vi "shiftregister&graphs.vi"() -> ()   [LabVIEW 2020]
panel:
  out "Waveform Graph":dbl[](graph)
  out "Waveform Chart":dbl(graph)
  in  "stop":bool
  out "Numeric 2":i64
  out "Numeric":i64
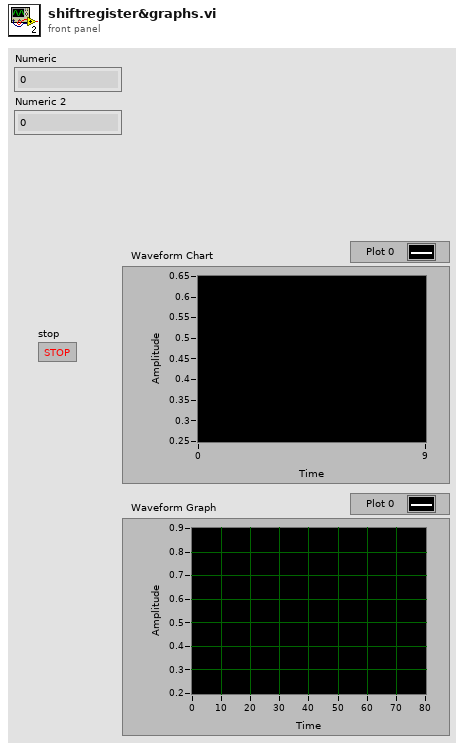
[diagram p1: front panel]
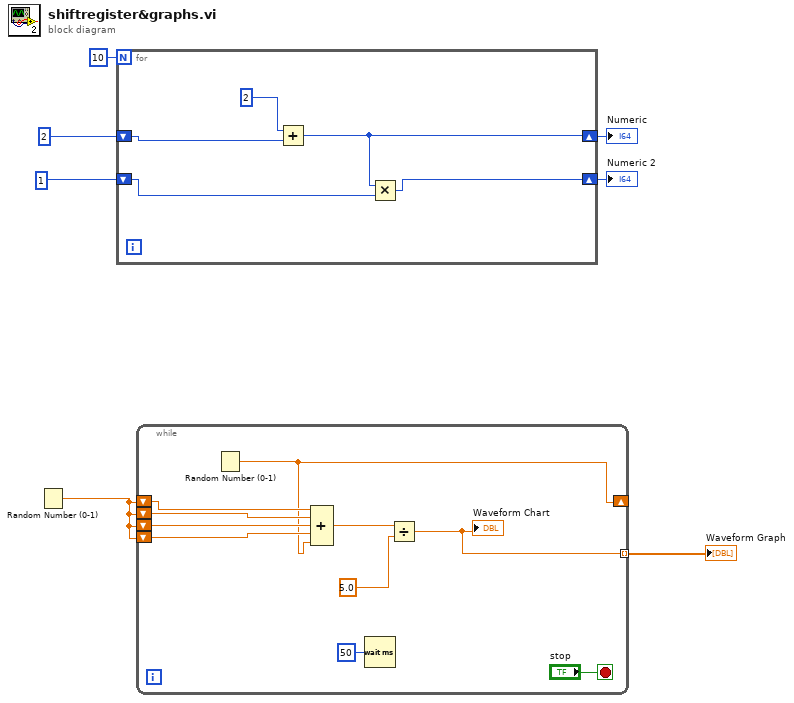
[diagram p0: block diagram]
diagram:
  n1 = Random Number (0-1)() -> (number: 0 to 1=w2:dbl)
  n2 = for {
    N: 10 -> [_]
    shift-right: [w8] -> w4
    shift-left: i64 2 -> [w12]
    shift-right: [w9] -> w3
    shift-left: i64 1 -> [w10]
    n3 = Add(x=i64 2, y=w12) -> (x+y=w8:i64)
    n4 = Multiply(x=w8, y=w10) -> (x*y=w9:i64)
  }
  "Numeric" <- w4
  "Numeric 2" <- w3
  n5 = while {
    shift-right: [w15] -> _
    shift-left: w2 -> [w21]
    shift-left: w2 -> [w20]
    shift-left: w2 -> [w19]
    shift-left: w2 -> [w18]
    tunnel: [w14] -> w1 mode=indexing
    stop <- "stop" stop-if-true
    n6 = Random Number (0-1)() -> (number: 0 to 1=w15:dbl)
    n7 = Compound Arithmetic op=ADD(w21, w20, w19, w18, w15) -> (w17:dbl)
    n8 = Wait (ms)(milliseconds to wait=u32 50) -> ()  [unwired: 1 out]
    n9 = Divide(x=w17, y=5.0) -> (x/y=w14:dbl)
    "Waveform Chart" <- w14
  }
  "Waveform Graph" <- w1
